vi "getToSortBy.vi"(8 "error in (no error)":errorcluster, 11 "BasicSortedNode in":refnum<class "BasicSortedNode.lvclass">) -> (0 "error out":errorcluster, 2 "ToSortBy":dbl, 3 "BasicSortedNode out":refnum<class "BasicSortedNode.lvclass">)   [LabVIEW 2009, in "BasicSortedNode.lvclass"]
doc: "Sets the value that is used to sort the list."
uses:
  BasicSortedNode.lvclass
  BasicSortedNode.lvclass/BasicSortedNode.ctl
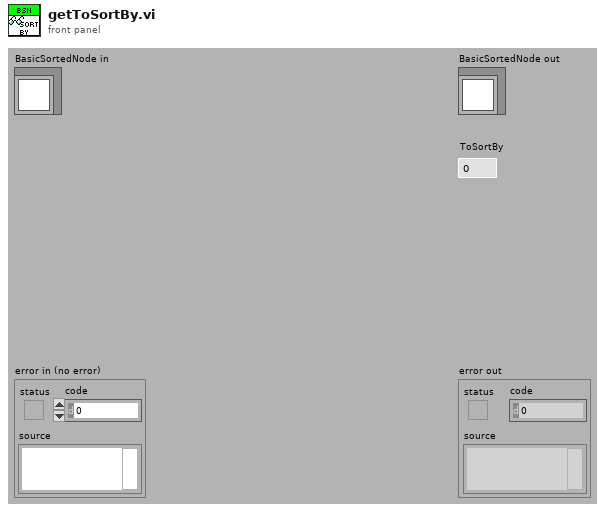
[diagram p1: front panel]
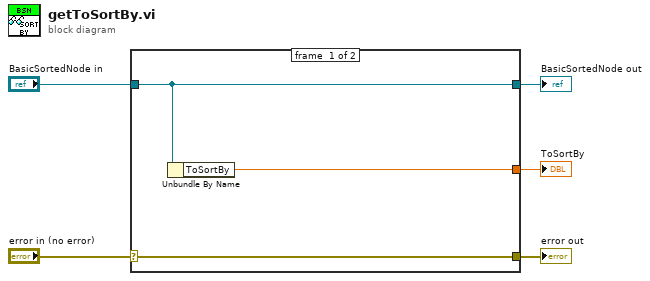
[diagram p0: block diagram]
diagram:
  n1 = case shown="No Error" "error in (no error)" {
    selector: "error in (no error)" -> [w8 w9]
    tunnel: [w8 w9] -> w4
    tunnel: [w7 w10] -> w2
    tunnel: "BasicSortedNode in" -> [w7 w10]
    tunnel: [w6 _] -> w1
    frame #0 {
      n2 = Unbundle By Name(w7) -> ("ToSortBy"=w6:dbl)
    }
    frame #1 {
    }
  }
  "error out" <- w4
  "BasicSortedNode out" <- w2
  "ToSortBy" <- w1
